vi "Toggle Switch.vi"(1 "Input":bool) -> (0 "Output":bool)   [LabVIEW 2016, in "2039lib.lvlib"]
uses:
  2039lib.lvlib
panel:
  out "Toggle":bool
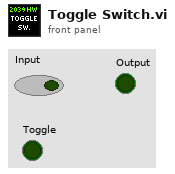
[diagram p1: front panel]
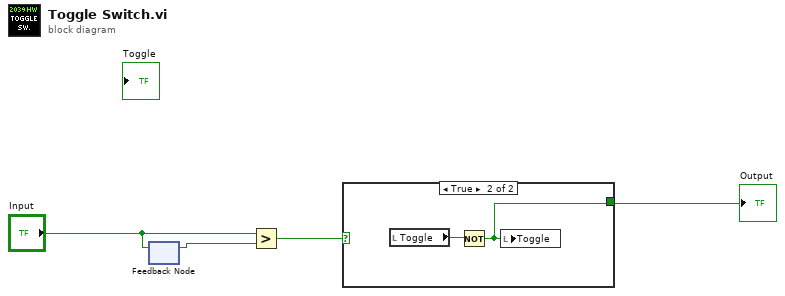
[diagram p0: block diagram]
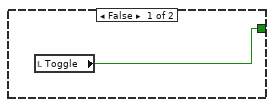
[diagram p2: hidden frame]
diagram:
  n1 = feedback-in #1("Input") -> ()
  n2 = feedback #1() -> (w4:bool)  [unwired: 1 in]
  n3 = Greater?(x="Input", y=w4) -> (0:w2:bool)
  n4 = case shown="True" w2 {
    tunnel: [w5 w6] -> w1
    frame False {
      n5 = local read "Toggle"() -> (w5:bool)
    }
    frame True {
      n6 = local read "Toggle"() -> (w7:bool)
      n7 = Not(x=w7) -> (.not. x?=w6:bool)
      n8 = local write "Toggle"(w6) -> ()
    }
  }
  "Output" <- w1
